vi "START EDIT ITEM.vi"(10 "USER/ITEM DATA TRANSFER IN":T2(array[cluster]), 11 "REFERENCES":T3) -> (3 "ITEM DATA OUT":T1)   [LabVIEW 2019]
uses:
  Controls/References Cluster.ctl
  <vilib>/userDefined/High Color/IMAQdx.ctl
  Controls/Custom Calendar/Custom Calendar.xctl
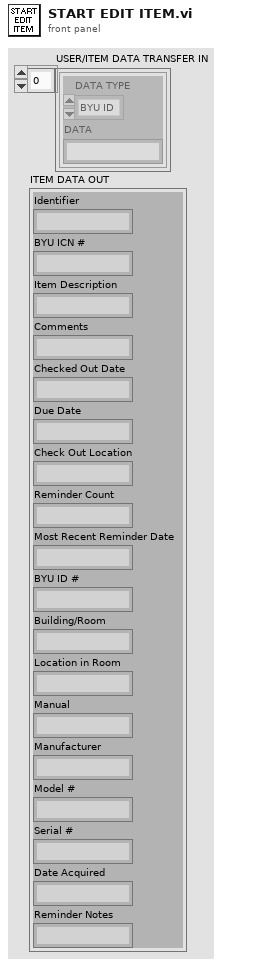
[diagram p1: front panel]
types:
  T1 = cluster{"Identifier":string, "BYU ICN #":string, "Item Description":string, "Comments":string, "Checked Out Date":string, "Due Date":string, "Check Out Location":string, "Reminder Count":string, "Most Recent Reminder Date":string, "BYU ID #":string, "Building/Room":string, "Location in Room":string, "Manual":string, "Manufacturer":string, "Model #":string, "Serial #":string, "Date Acquired":string, "Reminder Notes":string}
  T2 = cluster{"DATA TYPE":enum16{"BYU ID", "ME#/IDENTIFIER", "BYU ICN"}, "DATA":string}[]
  T3 = typedef "References Cluster.ctl" = cluster{"MAIN PAGES":refnum<vi>, "ADD/EDIT ITEM REFERENCES":cluster{"Identifier":refnum<vi>, "BYU ICN #":refnum<vi>, "Item Description":refnum<vi>, "Comments":refnum<vi>, "Checked Out Date":refnum<vi>, "Due Date":refnum<vi>, "Check Out Location":refnum<vi>, "Reminder Count":refnum<vi>, "Most Recent Reminder Date":refnum<vi>, "BYU ID #":refnum<vi>, "Building/Room":refnum<vi>, "Location in Room":refnum<vi>, "Manual":refnum<vi>, "Manufacturer":refnum<vi>, "Model #":refnum<vi>, "Serial #":refnum<vi>, "Date Acquired":refnum<vi>, "ADD/EDIT ITEM LABEL":refnum<vi>, "ARCHIVE ITEM":refnum<vi>, "Archive Item Inputs":refnum<vi>, "Reminder Notes":refnum<vi>, "DUPLICATE ITEM":refnum<vi>}, "ADD/EDIT USER REFERENCES":cluster{"BYU ID # (##-###-####)":refnum<vi>, "First Name":refnum<vi>, "Last Name":refnum<vi>, "Phone Number (###-###-####)":refnum<vi>, "Email":refnum<vi>, "Department":refnum<vi>, "Graduation Status":refnum<vi>, "Anticipated Graduation Year":refnum<vi>, "Credit Score":refnum<vi>, "Date Added":refnum<vi>, "Graduation Clearance Date":refnum<vi>, "Picture File Name":refnum<vi>, "ADD/EDIT USER LABEL":refnum<vi>, "Department Map":refnum<vi>, "Status Map":refnum<vi>, "Anticipated Graduation Year Map":refnum<vi>, "User Agreement":refnum<vi>, "User Comments":refnum<vi>, "Camera":refnum<vi>}, "RETURN ITEM REFERENCES":cluster{"Item or Person:":refnum<vi>, "Search Return Results":refnum<vi>, "What are you searching for?":refnum<vi>}, "SEARCH DATABASE REFERENCES":cluster{"What to Search For:":refnum<vi>, "Where to Search":refnum<vi>, "Column to Search In":refnum<vi>, "Column to Sort By":refnum<vi>, "Search Database Results":refnum<vi>, "Inventory Column Selector":refnum<vi>, "User Column Selector":refnum<vi>, "Inventory Archive Column Selector":refnum<vi>, "User Archive Column Selector":refnum<vi>, "Sales Tracking Column Selector":refnum<vi>, "Checked In Archive Column Selector":refnum<vi>, "Restore User":refnum<vi>, "Date Range":refnum<vi>, "Dates Less Than":refnum<vi>, "Dates Greater Than":refnum<vi>, "Search Print Receipt":refnum<vi>, "Edit Sale Description":refnum<vi>}, "USER ITEMS REFERENCES":cluster{"USER'S INFORMATION":refnum<vi>, "User's Checked Out Items":refnum<vi>, "User Info Comments":refnum<vi>, "SEE USER INFO COMMENTS":refnum<vi>}, "EDIT ITEMS REFERENCES":cluster{"New Check Out Location":refnum<vi>, "Items to Edit":refnum<vi>, "Edit Items Due Date":refnum<vi>, "New Reminder Notes":refnum<vi>, "New Item Description":refnum<vi>}, "CHECK OUT ITEMS REFERENCES":cluster{"Enter Item:":refnum<vi>, "Check Out Items Due Date":refnum<vi>, "Check Out Location":refnum<vi>, "Items to be Checked Out":refnum<vi>, "Possible Items":refnum<vi>, "Altered Item Description":refnum<vi>}, "TRANSFER ITEMS REFERENCES":cluster{"Search Parameter":refnum<vi>, "What to Match":refnum<vi>, "Matching Individuals":refnum<vi>, "Items to be Transferred":refnum<vi>}, "SETTINGS REFERENCES":cluster{"PSC Database Settings":refnum<vi>, "PSC Sales Item Spreadsheet":refnum<vi>}, "PSC SALES REFERENCES":cluster{"BYU ID CARD #":refnum<vi>, "Sale Description":refnum<vi>, "Scan or Enter Item Name":refnum<vi>, "Items to be Sold":refnum<vi>, "Grand Total":refnum<vi>, "Item List":refnum<vi>}}
  T4 = cluster{"Disposal Date":string, "Disposal Method":u16, "Auction # / Other":string, "Date Disposal Email Sent":string, "Disposal Notes":string}
  T5 = enum32{"IDLE", "ADD/EDIT USER", "ADD/EDIT ITEM", "RETURN ITEMS", "SEARCH DATABASE", "USER ITEMS", "CHECK OUT ITEMS", "EDIT ITEMS", "TRANSFER ITEMS", "PSC SALES", "ATRIUM", "INVENTORY TRACKING", "SETTINGS"}
  T6 = cluster{"Identifier":refnum<vi>, "BYU ICN #":refnum<vi>, "Item Description":refnum<vi>, "Comments":refnum<vi>, "Checked Out Date":refnum<vi>, "Due Date":refnum<vi>, "Check Out Location":refnum<vi>, "Reminder Count":refnum<vi>, "Most Recent Reminder Date":refnum<vi>, "BYU ID #":refnum<vi>, "Building/Room":refnum<vi>, "Location in Room":refnum<vi>, "Manual":refnum<vi>, "Manufacturer":refnum<vi>, "Model #":refnum<vi>, "Serial #":refnum<vi>, "Date Acquired":refnum<vi>, "ADD/EDIT ITEM LABEL":refnum<vi>, "ARCHIVE ITEM":refnum<vi>, "Archive Item Inputs":refnum<vi>, "Reminder Notes":refnum<vi>, "DUPLICATE ITEM":refnum<vi>}
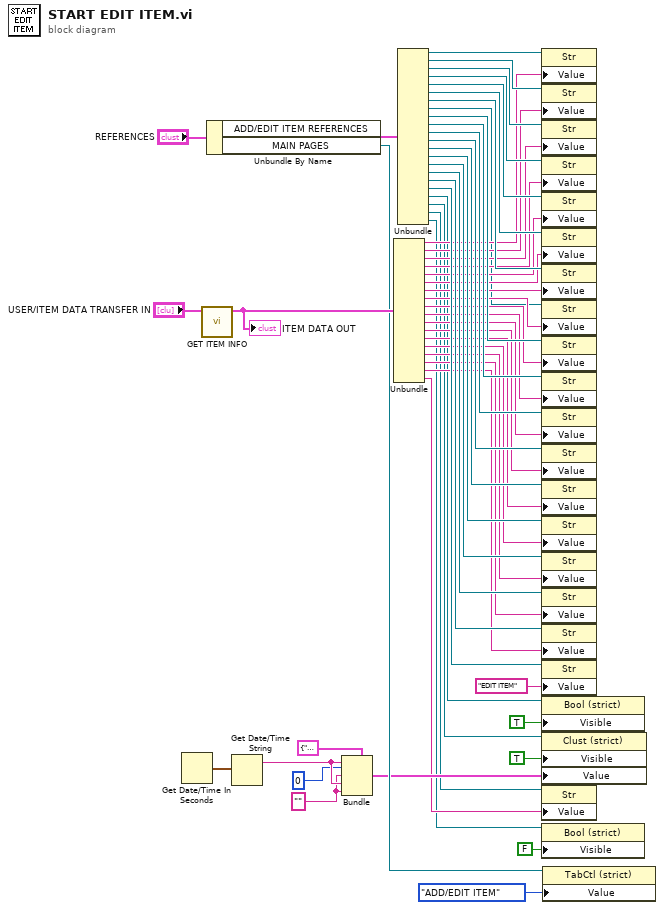
[diagram p0: block diagram]
diagram:
  w5 = "" ("Auction # / Other")
  n1 = Get Date/Time In Seconds() -> (seconds since 1Jan1904=w8:timestamp)
  n2 = call "GET ITEM INFO.vi"("USER/ITEM DATA TRANSFER IN"="USER/ITEM DATA TRANSFER IN") -> ("ITEM DATA OUT"=w14:T1)  [unwired: 10 in]
  "ITEM DATA OUT" <- w14
  n3 = Unbundle By Name("REFERENCES") -> ("ADD/EDIT ITEM REFERENCES"=w18:T6, "MAIN PAGES"=w13:refnum<vi>)
  n4 = Get Date/Time String(seconds (now)=w8) -> (date string=w7:string)  [unwired: 2 in, 1 out]
  n5 = Bundle(cluster=T4 {"Disposal Date"="", "Disposal Method"=0, "Auction # / Other"="", "Date Disposal Email Sent"="", "Disposal Notes"=""} ("Value"), "Disposal Date"=w7, "Disposal Method"=u16 0, "Auction # / Other"=w5, "Date Disposal Email Sent"=w7, "Disposal Notes"=w5) -> (w9:T4)
  n6 = Unbundle(w14) -> ("Identifier"=w38:string, "BYU ICN #"=w37:string, "Item Description"=w36:string, "Comments"=w35:string, "Checked Out Date"=w34:string, "Due Date"=w33:string, "Check Out Location"=w32:string, "Reminder Count"=w31:string, "Most Recent Reminder Date"=w30:string, "BYU ID #"=w29:string, "Building/Room"=w28:string, "Location in Room"=w27:string, "Manual"=w26:string, "Manufacturer"=w25:string, "Model #"=w24:string, "Serial #"=w23:string, "Date Acquired"=w22:string, "Reminder Notes"=w3:string)
  n7 = Unbundle(w18) -> ("Identifier"=w56:refnum<vi>, "BYU ICN #"=w55:refnum<vi>, "Item Description"=w54:refnum<vi>, "Comments"=w53:refnum<vi>, "Checked Out Date"=w52:refnum<vi>, "Due Date"=w51:refnum<vi>, "Check Out Location"=w50:refnum<vi>, "Reminder Count"=w16:refnum<vi>, "Most Recent Reminder Date"=w49:refnum<vi>, "BYU ID #"=w48:refnum<vi>, "Building/Room"=w47:refnum<vi>, "Location in Room"=w46:refnum<vi>, "Manual"=w45:refnum<vi>, "Manufacturer"=w44:refnum<vi>, "Model #"=w43:refnum<vi>, "Serial #"=w42:refnum<vi>, "Date Acquired"=w41:refnum<vi>, "ADD/EDIT ITEM LABEL"=w40:refnum<vi>, "ARCHIVE ITEM"=w21:refnum<vi>, "Archive Item Inputs"=w20:refnum<vi>, "Reminder Notes"=w4:refnum<vi>, "DUPLICATE ITEM"=w2:refnum<vi>)
  n8 = property class="Str"(reference=w56, "Value"=w38) -> ()  [unwired: 1 in, 2 out]
  n9 = property class="Str"(reference=w55, "Value"=w37) -> ()  [unwired: 1 in, 2 out]
  n10 = property class="Str"(reference=w54, "Value"=w36) -> ()  [unwired: 1 in, 2 out]
  n11 = property class="Str"(reference=w53, "Value"=w35) -> ()  [unwired: 1 in, 2 out]
  n12 = property class="Str"(reference=w52, "Value"=w34) -> ()  [unwired: 1 in, 2 out]
  n13 = property class="Str"(reference=w51, "Value"=w33) -> ()  [unwired: 1 in, 2 out]
  n14 = property class="Str"(reference=w50, "Value"=w32) -> ()  [unwired: 1 in, 2 out]
  n15 = property class="Str"(reference=w16, "Value"=w31) -> ()  [unwired: 1 in, 2 out]
  n16 = property class="Str"(reference=w49, "Value"=w30) -> ()  [unwired: 1 in, 2 out]
  n17 = property class="Str"(reference=w48, "Value"=w29) -> ()  [unwired: 1 in, 2 out]
  n18 = property class="Str"(reference=w47, "Value"=w28) -> ()  [unwired: 1 in, 2 out]
  n19 = property class="Str"(reference=w46, "Value"=w27) -> ()  [unwired: 1 in, 2 out]
  n20 = property class="Str"(reference=w45, "Value"=w26) -> ()  [unwired: 1 in, 2 out]
  n21 = property class="Str"(reference=w44, "Value"=w25) -> ()  [unwired: 1 in, 2 out]
  n22 = property class="Str"(reference=w43, "Value"=w24) -> ()  [unwired: 1 in, 2 out]
  n23 = property class="Str"(reference=w42, "Value"=w23) -> ()  [unwired: 1 in, 2 out]
  n24 = property class="Str"(reference=w41, "Value"=w22) -> ()  [unwired: 1 in, 2 out]
  n25 = property class="Str"(reference=w40, "Value"="EDIT ITEM" ("ADD/EDIT ITEM LABEL")) -> ()  [unwired: 1 in, 2 out]
  n26 = property class="Bool (strict)"(reference=w21, "Visible"=TRUE) -> ()  [unwired: 1 in, 2 out]
  n27 = property class="Clust (strict)"(reference=w20, "Visible"=TRUE, "Value"=w9) -> ()  [unwired: 1 in, 2 out]
  n28 = property class="Str"(reference=w4, "Value"=w3) -> ()  [unwired: 1 in, 2 out]
  n29 = property class="Bool (strict)"(reference=w2, "Visible"=FALSE) -> ()  [unwired: 1 in, 2 out]
  n30 = property class="TabCtl (strict)"(reference=w13, "Value"=T5."ADD/EDIT ITEM") -> ()  [unwired: 1 in, 2 out]
